vi "Periodic Tasks.vi"(8 "error in":errorcluster) -> ()   [LabVIEW 2013]
doc: "This VI runs in parallel to other tasks. It can contain as many user-defined periodic loops as you need. These can carry out PID or other sorts of timed response."
uses:
  <vilib>/Rock Robotics/SystemInterfaces/Utilities/FPGA_UtilitiesLED Source.ctl
  <vilib>/Rock Robotics/SystemInterfaces/Utilities/FPGA_UtilitiesLED State.ctl
  Robot Global Data.vi
panel:
  out "Distance":dbl
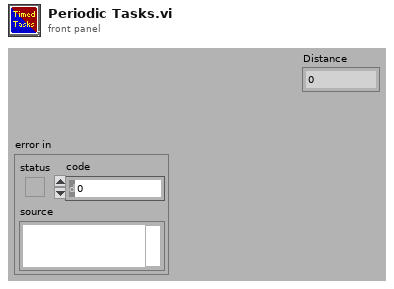
[diagram p1: front panel]
types:
  T1 = typedef "WPI_AnalogChannelDevRef.ctl" = cluster{"DevStatus":errorcluster, "Analog Module":T2, "Analog Channel":T3}
  T2 = typedef "FPGA_TypedefAnalogModule.ctl" = enum16{"Analog Module 1", "Analog Module 2"}
  T3 = typedef "FPGA_AIChannel.ctl" = enum8{"AI 1", "AI 2", "AI 3", "AI 4", "AI 5", "AI 6", "AI 7", "AI 8", "Invalid"}
  T4 = typedef "WPI_JoystickButtonState.ctl" = cluster{"Button 1":bool, "Button 2":bool, "Button 3":bool, "Button 4":bool, "Button 5":bool, "Button 6":bool, "Button 7":bool, "Button 8":bool, "Button 9":bool, "Button 10":bool, "Button 11":bool, "Button 12":bool}
  T5 = typedef "WPI_DigitalInputDevRef.ctl" = cluster{"DevStatus":errorcluster, "DIO Channel":T6, "Digital Module":T7}
  T6 = typedef "FPGA_DIOChannel.ctl" = enum8{"DIO 1", "DIO 2", "DIO 3", "DIO 4", "DIO 5", "DIO 6", "DIO 7", "DIO 8", "DIO 9", "DIO 10", "DIO 11", "DIO 12", "DIO 13", "DIO 14", "Invalid"}
  T7 = typedef "FPGA_TypedefDigitalModule.ctl" = enum16{"Digital Module 1", "Digital Module 2"}
  T8 = typedef "WPI_EncoderDevRef.ctl" = cluster{"DevStatus":errorcluster, "EncoderIndex":T9, "CounterIndex":T10, "DistancePerCount":dbl, "Decoding Type":T11}
  T9 = typedef "FPGA_EncoderIdx.ctl" = enum8{"Enc 0", "Enc 1", "Enc 2", "Enc 3", "Invalid"}
  T10 = typedef "FPGA_CounterCtrSystemIndex.ctl" = enum8{"Ctr 0", "Ctr 1", "Ctr 2", "Ctr 3", "Ctr 4", "Ctr 5", "Ctr 6", "Ctr 7", "Invalid"}
  T11 = typedef "WPI_EncoderType.ctl" = enum16{"1x", "2x", "4x"}
  T12 = typedef "FPGA_UtilitiesLED State.ctl" = enum16{"Off", "On", "Toggle"}
  T13 = typedef "FPGA_UtilitiesLED Source.ctl" = enum16{"User LED", "FPGA LED"}
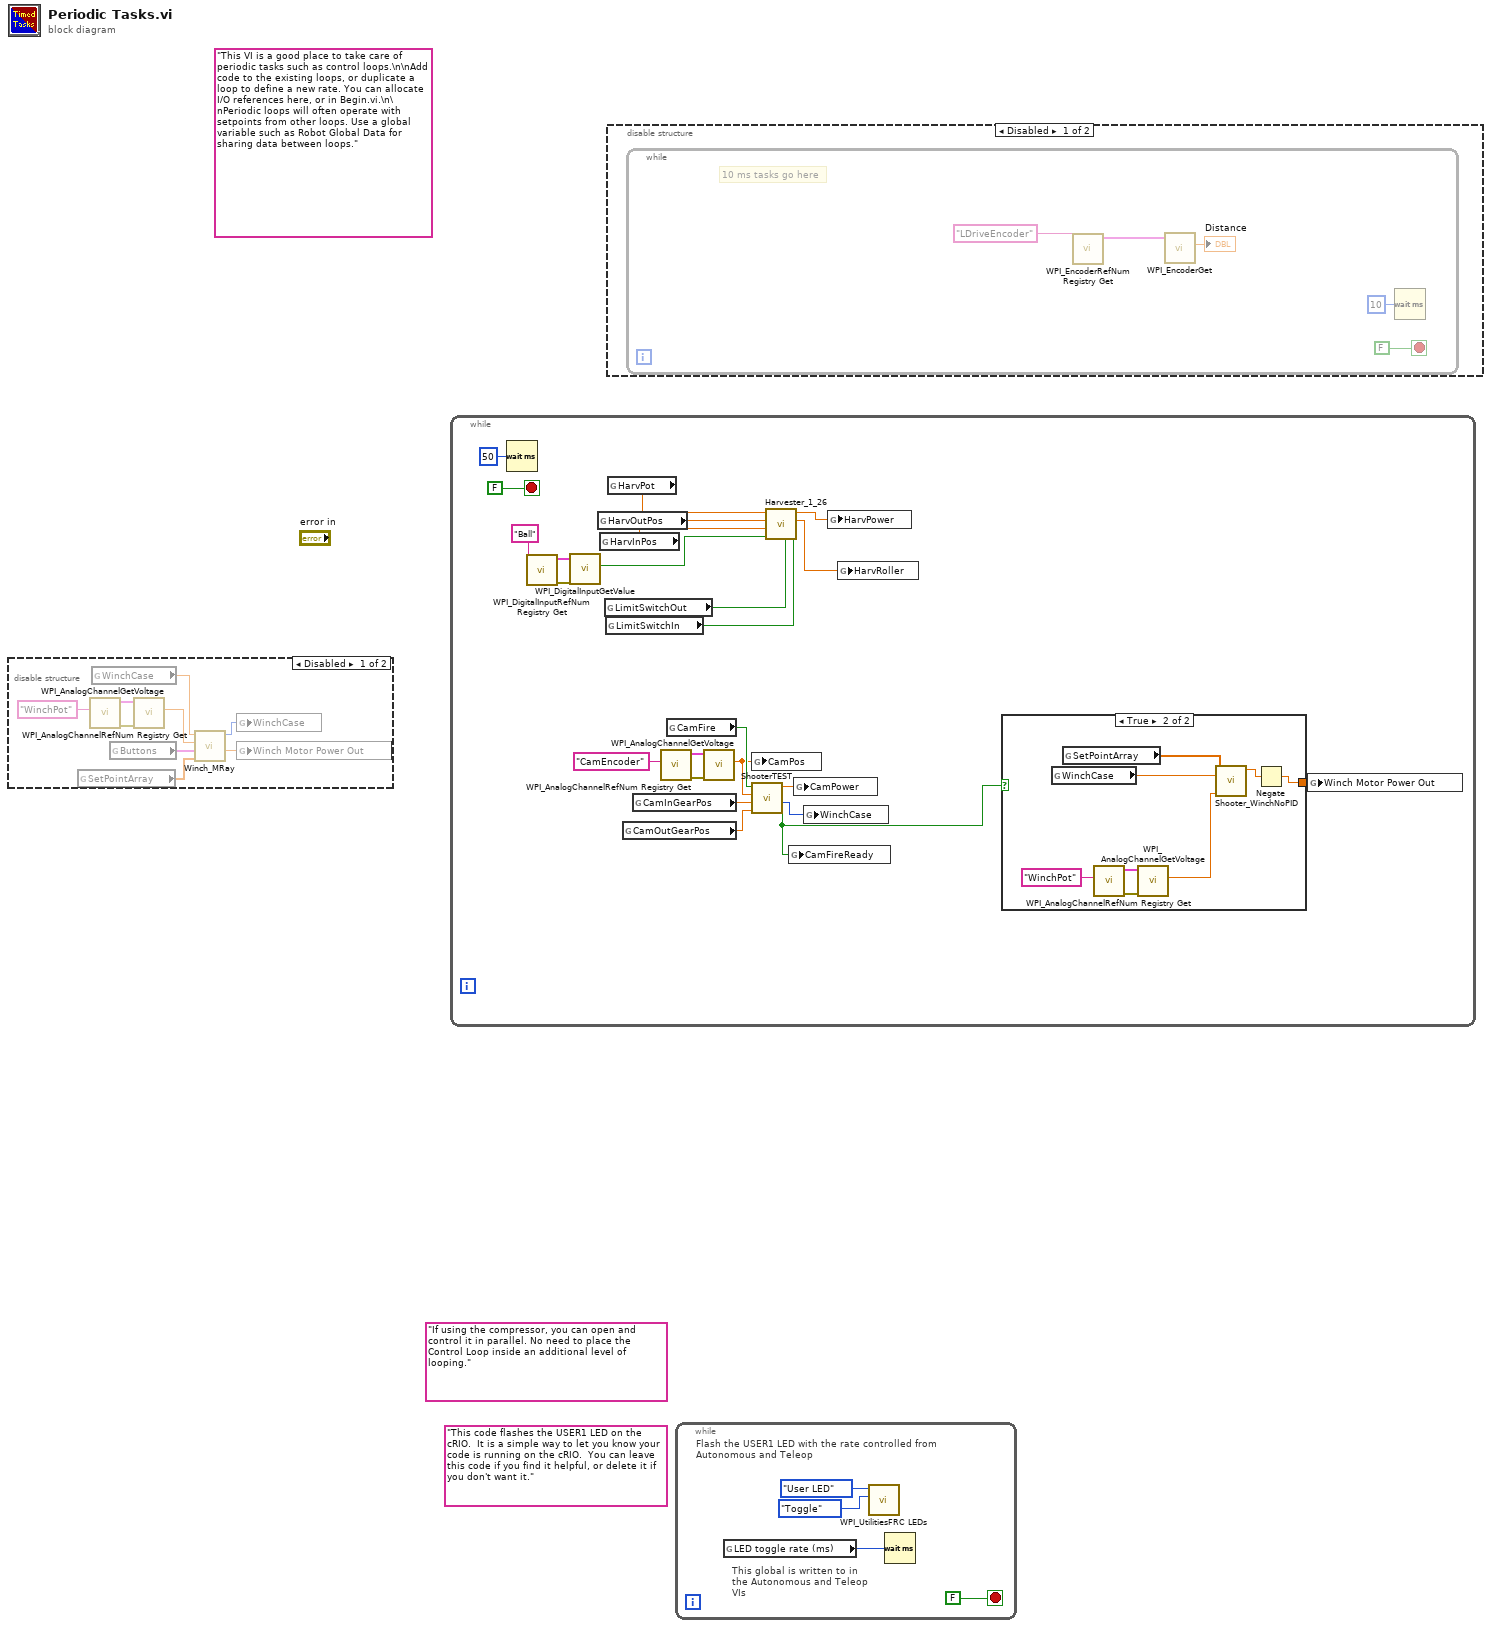
[diagram p0: block diagram]
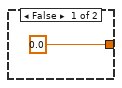
[diagram p4: hidden frame]
diagram:
  (unwired) "If using the compressor, you can open and control it in parallel. No need to place the Control Loop inside an additional level of looping."
  (unwired) "This code flashes the USER1 LED on the cRIO.  It is a simple way to let you know your code is running on the cRIO.  You can leave this code if you find it helpful, or delete it if you don't want it."
  (unwired) "This VI is a good place to take care of periodic tasks such as control loops.\n\nAdd code to the existing loops, or duplicate a loop to define a new rate. You can allocate I/O references here, or in Begin.vi.\n\nPeriodic loops will often operate with setpoints from other loops. Use a global variable such as Robot Global Data for sharing data between loops."
  n1 = disable-structure shown="Disabled" {
    frame Disabled {
      n2 = global read "Robot Global Data.vi" "SetPointArray"() -> (w5:dbl[])
      n3 = call <vilib>:"WPI_AnalogChannelRefNum Registry Get.vi"("refnum name"="WinchPot") -> ("error out"=w8:errorcluster, "AIDeviceRef"=w7:T1)  [unwired: 9 in]
      n4 = global read "Robot Global Data.vi" "WinchCase"() -> (w1:dbl)
      n5 = global read "Robot Global Data.vi" "Buttons"() -> (w6:T4)
      n6 = call <vilib>:"WPI_AnalogChannelGetVoltage.vi"("error in (no error)"=w8, "AIDeviceRef"=w7) -> ("Voltage"=w3:dbl)  [unwired: 7 in, 2 out]
      n7 = call "Winch_MRay.vi"("Setpoints"=w5, "Buttons"=w6, "Current POT"=w3, "Winch State"=w1) -> ("Winch Out"=w4:dbl, "Winch State"=w2:i32)  [unwired: 6 in]
      n8 = global write "Robot Global Data.vi" "WinchCase"(w2) -> ()
      n9 = global write "Robot Global Data.vi" "Winch Motor Power Out"(w4) -> ()
    }
    frame Enabled {
    }
  }
  n10 = while {
    stop <- FALSE stop-if-true
    n11 = Wait (ms)(milliseconds to wait=u32 50) -> ()  [unwired: 1 out]
    n12 = call <vilib>:"WPI_DigitalInputRefNum Registry Get.vi"("refnum name"="Ball") -> ("error out"=w15:errorcluster, "DigitalInputDevRef"=w14:T5)  [unwired: 9 in]
    n13 = call <vilib>:"WPI_DigitalInputGetValue.vi"("error in (no error)"=w15, "DigitalInputDevRef"=w14) -> ("Value"=w13:bool)  [unwired: 7 in, 2 out]
    n14 = global read "Robot Global Data.vi" "HarvOutPos"() -> (w21:dbl)
    n15 = global read "Robot Global Data.vi" "HarvInPos"() -> (w20:dbl)
    n16 = global read "Robot Global Data.vi" "LimitSwitchOut"() -> (w19:bool)
    n17 = global read "Robot Global Data.vi" "LimitSwitchIn"() -> (w18:bool)
    n18 = global read "Robot Global Data.vi" "HarvPot"() -> (w22:dbl)
    n19 = global read "Robot Global Data.vi" "CamOutGearPos"() -> (w29:dbl)
    n20 = global read "Robot Global Data.vi" "CamInGearPos"() -> (w30:dbl)
    n21 = call <vilib>:"WPI_AnalogChannelRefNum Registry Get.vi"("refnum name"="CamEncoder") -> ("error out"=w26:errorcluster, "AIDeviceRef"=w25:T1)  [unwired: 9 in]
    n22 = global read "Robot Global Data.vi" "CamFire"() -> (w31:bool)
    n23 = call <vilib>:"WPI_AnalogChannelGetVoltage.vi"("error in (no error)"=w26, "AIDeviceRef"=w25) -> ("Voltage"=w24:dbl)  [unwired: 7 in, 2 out]
    n24 = global write "Robot Global Data.vi" "CamPos"(w24) -> ()
    n25 = call "ShooterTEST.vi"("OutGearPos"=w29, "InGearPos"=w30, "Pot"=w24, "Fire"=w31) -> ("There?"=w11:bool, "WinchCase"=w10:i32, "Power"=w28:dbl)  [unwired: 5 in]
    n26 = call "Harvester_1_26.vi"("LimitSwitchIn"=w18, "LimitSwitchOut"=w19, "BallInHarv"=w13, "HarvInPos"=w20, "HarvOutPos"=w21, "HarvPot"=w22) -> ("HarvRoller"=w17:dbl, "HarvPower"=w16:dbl)  [unwired: 4 in]
    n27 = global write "Robot Global Data.vi" "CamFireReady"(w11) -> ()
    n28 = global write "Robot Global Data.vi" "CamPower"(w28) -> ()
    n29 = global write "Robot Global Data.vi" "WinchCase"(w10) -> ()
    n30 = global write "Robot Global Data.vi" "HarvPower"(w16) -> ()
    n31 = global write "Robot Global Data.vi" "HarvRoller"(w17) -> ()
    n32 = case shown="True" w11 {
      tunnel: [0.0 ("Winch Motor Power Out") w35] -> w23
      frame False {
      }
      frame True {
        n33 = global read "Robot Global Data.vi" "WinchCase"() -> (w37:dbl)
        n34 = global read "Robot Global Data.vi" "SetPointArray"() -> (w39:dbl[])
        n35 = call <vilib>:"WPI_AnalogChannelRefNum Registry Get.vi"("refnum name"="WinchPot") -> ("error out"=w41:errorcluster, "AIDeviceRef"=w42:T1)  [unwired: 9 in]
        n36 = call <vilib>:"WPI_AnalogChannelGetVoltage.vi"("error in (no error)"=w41, "AIDeviceRef"=w42) -> ("Voltage"=w38:dbl)  [unwired: 7 in, 2 out]
        n37 = call "Shooter_WinchNoPID.vi"("Winch Pot Location"=w38, "selectedCase"=w37, "SetPointArray"=w39) -> ("Winch Motor Power Out"=w36:dbl)  [unwired: 8 in]
        n38 = Negate(x=w36) -> (-x=w35:dbl)
      }
    }
    n39 = global write "Robot Global Data.vi" "Winch Motor Power Out"(w23) -> ()
  }
  n40 = disable-structure shown="Disabled" {
    frame Disabled {
      n41 = while {
        stop <- FALSE stop-if-true
        # "10 ms tasks go here"
        n42 = call <vilib>:"WPI_EncoderRefNum Registry Get.vi"("refnum name"="LDriveEncoder") -> ("EncoderDevRef"=w43:T8)  [unwired: 9 in, 1 out]
        n43 = call <vilib>:"WPI_EncoderGet.vi"("EncoderDevRef"=w43) -> ("Distance"=→"Distance":dbl)  [unwired: 5 in, 5 out]
        n44 = Wait (ms)(milliseconds to wait=u32 10) -> ()  [unwired: 1 out]
      }
    }
    frame Enabled {
    }
  }
  n45 = while {
    stop <- FALSE stop-if-true
    # "This global is written to in the Autonomous and Teleop VIs"
    # "Flash the USER1 LED with the rate controlled from Autonomous and Teleop"
    n46 = global read "Robot Global Data.vi" "LED toggle rate (ms)"() -> (w48:u32)
    n47 = call <vilib>:"WPI_UtilitiesFRC LEDs.vi"("State"=FPGA_UtilitiesLED_State."Toggle", "LED Type"=FPGA_UtilitiesLED_Source."User LED") -> ()  [unwired: 1 in, 9 out]
    n48 = Wait (ms)(milliseconds to wait=w48) -> ()  [unwired: 1 out]
  }
